vi "SBG_Ellipse_case_select_n_buffer (SubVI).vi"(6 "new data in":string, 7 "buffer data in":string) -> (0 "case_selector":string, 1 "data out":string, 2 "msg_id":string, 4 "Data skipped":bool)   [LabVIEW 2017]
doc: "Filters out unwanted/unneccesary data packets, and sends remaining buffer to case structure to be read. Looks for start bytes FF5A (hex) and consecutive identifiers 03 (Acceleration and Internal Temperature), 13 (Odometer velocity), and 24 (Pressure). Additionally, throws out data that is not readable."
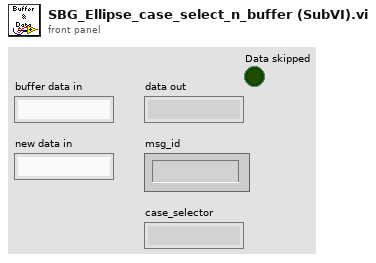
[diagram p1: front panel]
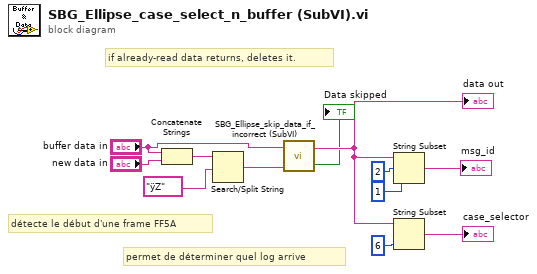
[diagram p0: block diagram]
diagram:
  # "if already-read data returns, deletes it."
  # "permet de déterminer quel log arrive"
  # "détecte le début d'une frame FF5A"
  n1 = Concatenate Strings("buffer data in", "new data in") -> (w3:string)
  n2 = Search/Split String(string=w3, search string/char (-)="ÿZ") -> (match + rest of string=w2:string)  [unwired: 1 in, 2 out]
  n3 = call "SBG_Ellipse_skip_data_if_incorrect (SubVI).vi"("String"=w2, "result string in"="buffer data in") -> ("Data skipped"=→"Data skipped":bool, "result string out"=w6:string)  [unwired: 1 in]
  "data out" <- w6
  n4 = String Subset(string=w6, offset (0)=2, length (rest)=1 ("length (rest)")) -> (substring=→"msg_id":string)
  n5 = String Subset(string=w6, length (rest)=6 ("length (len. of substring)")) -> (substring=→"case_selector":string)  [unwired: 1 in]
